vi "Generate CSRF.vi"(10 "Token ID":string, 11 "Key":string) -> (3 "Generated Token":string)   [LabVIEW 2020, in "HTTP Server.lvlib"]
uses:
  HTTP Server.lvlib
  lv-web-crypto/lv-crypto/Crypto/Hashes/SHA-256/SHA-256.lvclass
  lv-web-crypto/lv-base64/Variant.ctl
  lv-web-crypto/lv-base64/Base64.lvlib
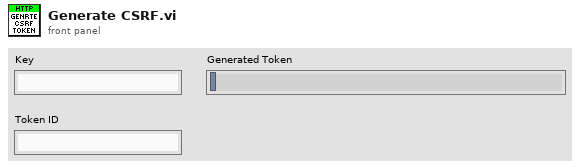
[diagram p1: front panel]
types:
  T1 = typedef "Base64.lvlib/Variant.ctl" = enum16{"Base64", "Base64-URL"}
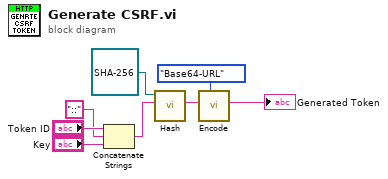
[diagram p0: block diagram]
diagram:
  n1 = Concatenate Strings("Token ID", "::" ("string"), "Key") -> (w5:string)
  n2 = call-dynamic "Hash.vi"("Message"=w5, "SHA-256 in"=refnum<class "SHA-256.lvclass"> refnum ("Crypto.lvlib:SHA-256.lvclass")) -> ("Hash"=w3:string)  [unwired: 7 in, 2 out]
  n3 = call "Encode.vi"("Variant (Base64)"=Variant."Base64-URL", "string in (not encoded)"=w3) -> ("string out (base64-encoded)"=→"Generated Token":string)  [unwired: 8 in, 1 out]
